vi "Check_In_Range.vi"(8 "error in (no error)":errorcluster, 10 "MeasurementVoltage":dbl, 11 "instrument handle":refnum<k15>) -> (0 "error out":errorcluster, 2 "Out of Range":bool)   [LabVIEW 2021, in "niDMM.lvclass"]
uses:
  niDMM.lvclass
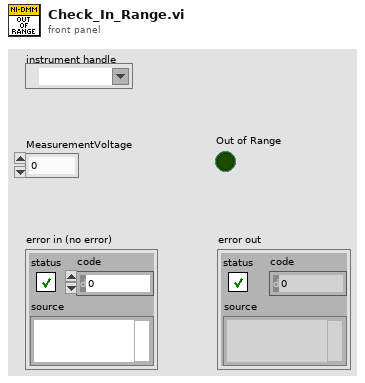
[diagram p1: front panel]
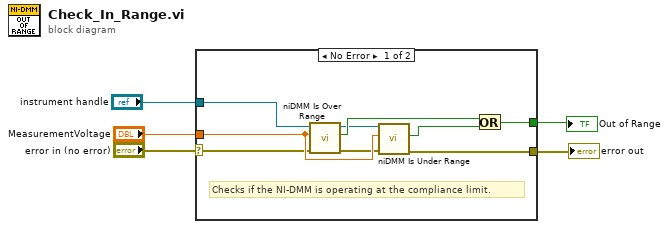
[diagram p0: block diagram]
diagram:
  n1 = case shown="No Error" "error in (no error)" {
    selector: "error in (no error)" -> [w8 w15]
    tunnel: [w12 _] -> w5
    tunnel: "MeasurementVoltage" -> [w11 _]
    tunnel: [w9 w15] -> w3
    tunnel: "instrument handle" -> [w6 _]
    frame No Error {
      # "Checks if the NI-DMM is operating at the compliance limit."
      n2 = call <instrlib>:"niDMM Is Over Range.vi"("error in (no error)"=w8, "Measurement"=w11, "instrument handle"=w6) -> ("error out"=w10:errorcluster, "Over Range?"=w13:bool, "instrument handle out"=w7:refnum<k15>)  [unwired: 6 in]
      n3 = call <instrlib>:"niDMM Is Under Range.vi"("error in (no error)"=w10, "Measurement"=w11, "instrument handle"=w7) -> ("error out"=w9:errorcluster, "Under Range?"=w14:bool)  [unwired: 6 in, 1 out]
      n4 = Or(x=w13, y=w14) -> (x .or. y?=w12:bool)
    }
    frame Error {
    }
  }
  "error out" <- w3
  "Out of Range" <- w5
